vi "About LabVIEW Open Source Project.vi"() -> ()   [LabVIEW 2013]
panel:
  out "Explore the project on GitHub":string
  # "LabVIEW Open Source Project\nReuse libraries for the Community"
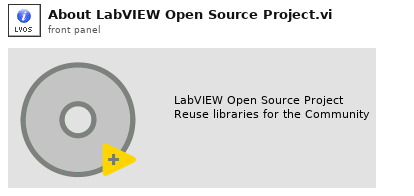
[diagram p1: front panel]
types:
  T1 = enum32{"Invalid", "Standard", "Closed", "Hidden", "Minimized", "Maximized"}
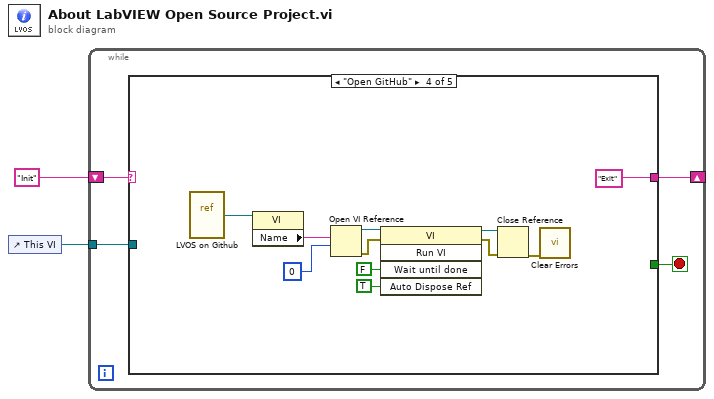
[diagram p0: block diagram]
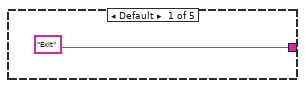
[diagram p2: hidden frame]
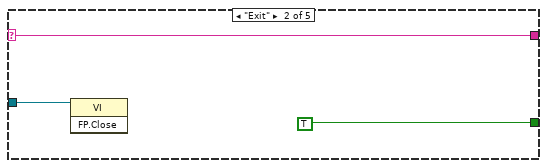
[diagram p3: hidden frame]
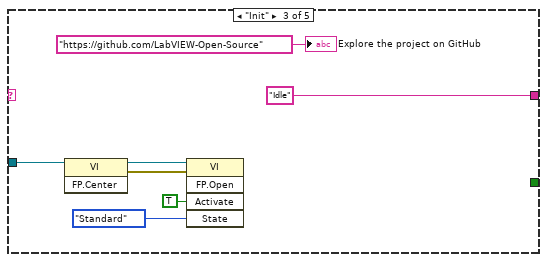
[diagram p4: hidden frame]
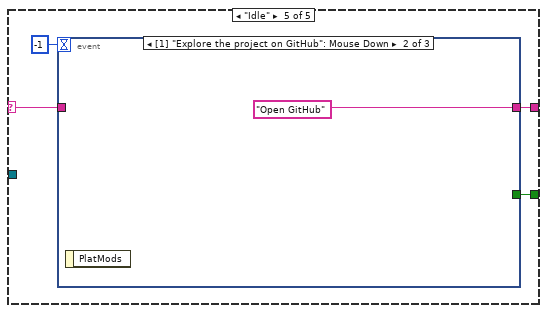
[diagram p5: hidden frame]
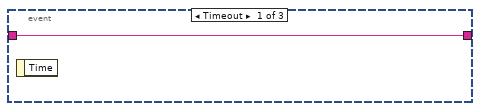
[diagram p6: hidden frame]
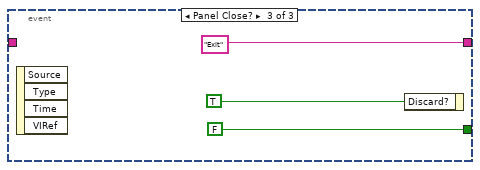
[diagram p7: hidden frame]
diagram:
  n1 = control-ref of="This VI"() -> (w1:refnum<vi>)
  n2 = while {
    shift-right: [w5] -> _
    shift-left: "Init" -> [w4]
    tunnel: w1 -> [w3]
    stop <- w6 stop-if-true
    n3 = case shown="\"Open GitHub\"" w4 {
      selector: w4 -> [_ w9 _ _ w29]
      tunnel: [_ TRUE _ _ w31] -> w6
      tunnel: ["Exit" w9 "Idle" "Exit" w30] -> w5
      tunnel: w3 -> [_ w8 w16 _ _]
      frame Default {
      }
      frame "Exit" {
        n4 = invoke class="VI" method="FP.Close"(reference=w8) -> ()  [unwired: 2 in, 3 out]
      }
      frame "Init" {
        n5 = invoke class="VI" method="FP.Center"(reference=w16) -> (reference out=w15:refnum<vi>, error out=w12:errorcluster)  [unwired: 2 in, 1 out]
        n6 = invoke class="VI" method="FP.Open"(reference=w15, error in=w12, "Activate"=TRUE ("Activate?"), "State"=T1."Standard") -> ()  [unwired: 1 in, 5 out]
        "Explore the project on GitHub" <- "https://github.com/LabVIEW-Open-Source" ("Explore the project on GitHub")
      }
      frame "Open GitHub" {
        n7 = vi-ref "LVOS on Github.vi"() -> (w27:refnum<vi>)
        n8 = property class="VI"(reference=w27) -> ("Name"=w26:string)  [unwired: 1 in, 2 out]
        n9 = Open VI Reference(vi path=w26, options=0) -> (vi reference=w24:refnum<vi>, error out=w21:errorcluster)  [unwired: 4 in]
        n10 = invoke class="VI" method="Run VI"(reference=w24, error in=w21, "Wait until done"=FALSE ("Wait Until Done"), "Auto Dispose Ref"=TRUE ("Auto Dispose Reference")) -> (reference out=w20:refnum<vi>, error out=w19:errorcluster)  [unwired: 1 in, 3 out]
        n11 = Close Reference(reference=w20, error in (no error)=w19) -> (error out=w18:errorcluster)
        n12 = call <vilib>:"Clear Errors.vi"("error in (no error)"=w18) -> ()  [unwired: 6 in, 1 out]
      }
      frame "Idle" {
        n13 = event shown="[1] \"Explore the project on GitHub\": Mouse Down" {
          selector: _ -> [_ _ _]
          dyn-events: _ -> [_ _ _]
          timeout: -1 -> [_ _ _]
          tunnel: [_ _ FALSE ("Discard?")] -> w31
          tunnel: w29 -> [w33 _ _]
          tunnel: [w33 "Open GitHub" "Exit"] -> w30
          event Timeout {
            n14 = event-data() -> ()  [unwired: 1 in, 1 out]
          }
          event "Explore the project on GitHub": Mouse Down {
            n15 = event-data() -> ()  [unwired: 1 in, 1 out]
          }
          event Panel Close? {
            n16 = event-data() -> ()  [unwired: 1 in, 4 out]
            n17 = event-data("Discard?"=TRUE) -> ()  [unwired: 1 in, 1 out]
          }
        }
      }
    }
  }
